vi "parseReadPIDParametersResponse.vi"(8 "error in (no error)":errorcluster, 10 "DynamicFrameParser":refnum<class "DynamicFrameParser.lvclass">, 11 "FAILC in":refnum<class "FAILC.lvclass">) -> (0 "error out":errorcluster, 3 "FAILC out":refnum<class "FAILC.lvclass">)   [LabVIEW 2016, in "RTFAILC.lvlib" / "FAILC.lvclass"]
uses:
  FAILC.lvclass
  Common_RT_Modbus/DynamicFrameParser/DynamicFrameParser.lvclass
  Common_RT_Modbus/DataTypes/ExceptionCodes.ctl
  FAILC.lvclass/FAILC.ctl
  Common_RT_Modbus/RTModbus.lvlib
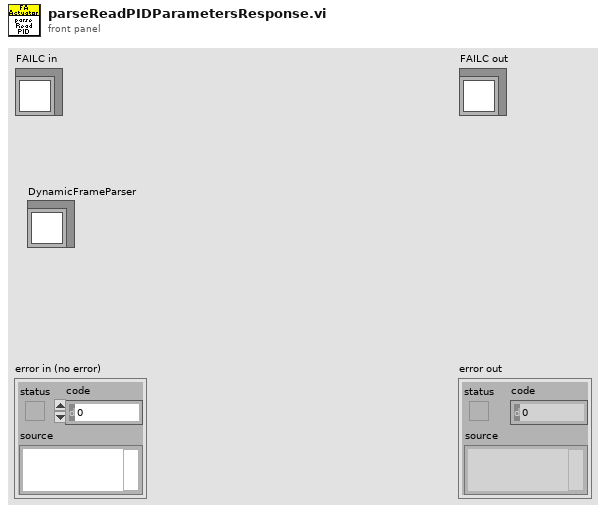
[diagram p1: front panel]
types:
  T1 = typedef "RTModbus.lvlib/ExceptionCodes.ctl" = u16
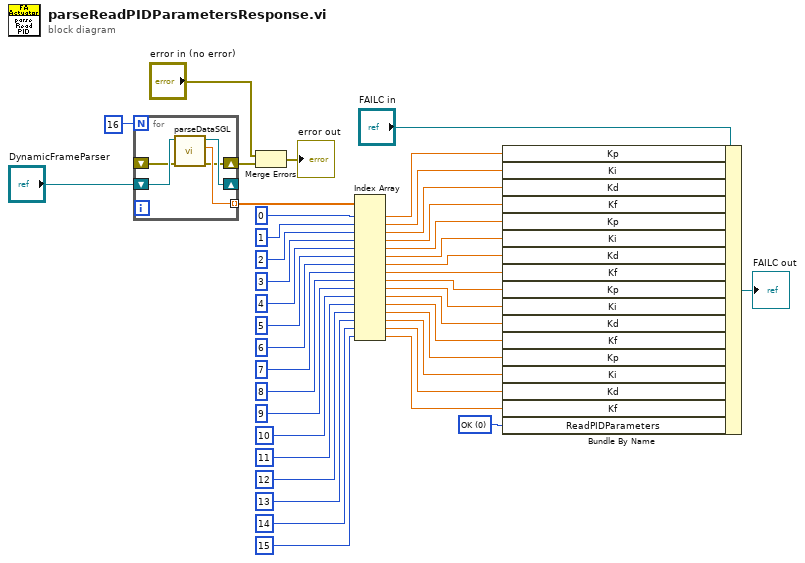
[diagram p0: block diagram]
diagram:
  w39 = T1 0 items=["OK", "IllegalFunction", "IllegalDataAddress", "IllegalDataValue", "SlaveDeviceFailure", "Acknowledge", "SlaveDeviceBusy", "NegativeAcknowledge", "MemoryParityError", "GatewayPathUnavailable", "GatewayTargetDeviceFailedToRespond"] ("FAData.FAResponses.PIDParameters")
  n1 = for {
    N: 16 -> [_]
    shift-right: [w45] -> _
    shift-left: "DynamicFrameParser" -> [w46]
    tunnel: [w44] -> w37 mode=indexing
    shift-right: [w42] -> w3
    shift-left: _ -> [w43]
    n2 = call "parseDataSGL.vi"("error in (no error)"=w43, "FrameParser in"=w46) -> ("error out"=w42:errorcluster, "Data"=w44:sgl, "FrameParser out"=w45:refnum<class "DynamicFrameParser.lvclass">)  [unwired: 7 in]
  }
  n3 = Merge Errors("error in (no error)", w3) -> (→"error out":errorcluster)
  n4 = Index Array(array=w37, index #1=0 ("index"), index #2=1 ("index"), index #3=2 ("index"), index #4=3 ("index"), index #5=4 ("index"), index #6=5 ("index"), index #7=6 ("index"), index #8=7 ("index"), index #9=8 ("index"), index #10=9 ("index"), index #11=10 ("index"), index #12=11 ("index"), index #13=12 ("index"), index #14=13 ("index"), index #15=14 ("index"), index #16=15 ("index")) -> (element #1=w20:sgl, element #2=w19:sgl, element #3=w18:sgl, element #4=w17:sgl, element #5=w16:sgl, element #6=w15:sgl, element #7=w14:sgl, element #8=w13:sgl, element #9=w12:sgl, element #10=w11:sgl, element #11=w10:sgl, element #12=w9:sgl, element #13=w8:sgl, element #14=w7:sgl, element #15=w6:sgl, element #16=w5:sgl)
  n5 = Bundle By Name(cluster="FAILC in", "Kp"=w20, "Ki"=w19, "Kd"=w18, "Kf"=w17, "Kp"=w16, "Ki"=w15, "Kd"=w14, "Kf"=w13, "Kp"=w12, "Ki"=w11, "Kd"=w10, "Kf"=w9, "Kp"=w8, "Ki"=w7, "Kd"=w6, "Kf"=w5, "ReadPIDParameters"=w39) -> (→"FAILC out":refnum<class "FAILC.lvclass">)
